vi "Picture Ring to Grid.vi"(11 "Selection Grid":T5) -> (1 "Valid":bool, 2 "Grid Summary":T4, 3 "Map":map{T1, T2}(c390))   [LabVIEW 2019, in "Grassfire Algorithm.lvclass"]
doc: "From the Start Grid of just the picture ring array, calculate where the start and end are."
uses:
  Grassfire Algorithm.lvclass
  Selection Grid Cell--array.ctl
  Selection--picture ring.ctl
  Grid Summary--cluster.ctl
  Index Column Row--cluster.ctl
  Solution Grid Cell Private--cluster.ctl
  Solution--picture ring.ctl
panel:
  out "1 End":bool
  out "1 Start":bool
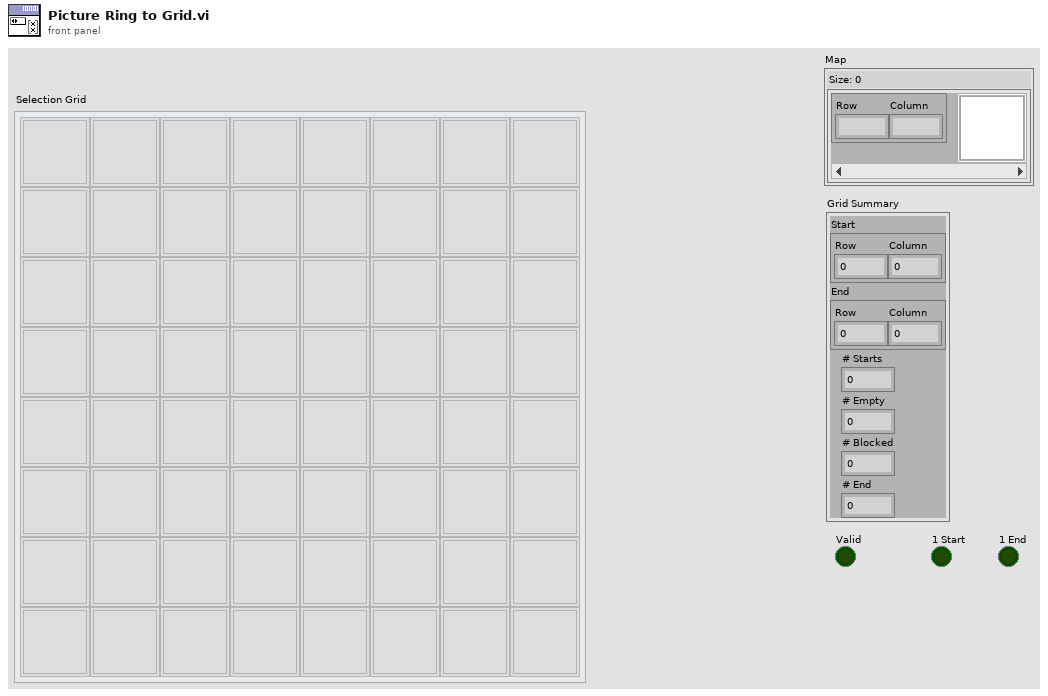
[diagram p1: front panel]
types:
  T1 = typedef "Grassfire Algorithm.lvclass/Index Column Row--cluster.ctl" = cluster{"Row":i32, "Column":i32}
  T2 = typedef "Grassfire Algorithm.lvclass/Solution Grid Cell Private--cluster.ctl" = cluster{"Picture":T3, "Value":dbl}
  T3 = typedef "Grassfire Algorithm.lvclass/Solution--picture ring.ctl" = i64
  T4 = typedef "Grassfire Algorithm.lvclass/Grid Summary--cluster.ctl" = cluster{"Start":T1, "End":T1, "# Starts":i32, "# Empty":i32, "# Blocked":i32, "# End":i32}
  T5 = typedef "Grassfire Algorithm.lvclass/Selection Grid Cell--array.ctl" = cluster{"Grid Value":T6}[][]
  T6 = typedef "Grassfire Algorithm.lvclass/Selection--picture ring.ctl" = i64
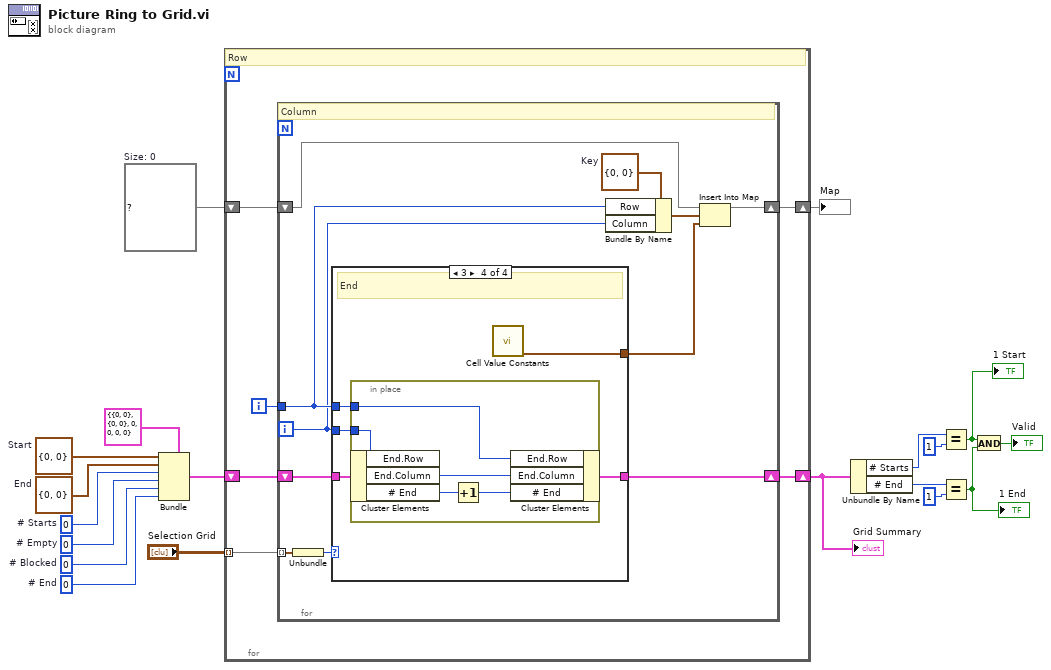
[diagram p0: block diagram]
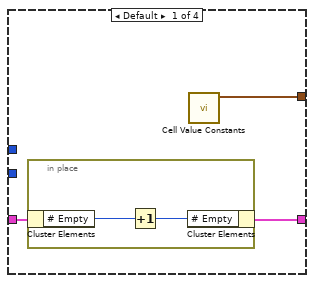
[diagram p2: hidden frame]
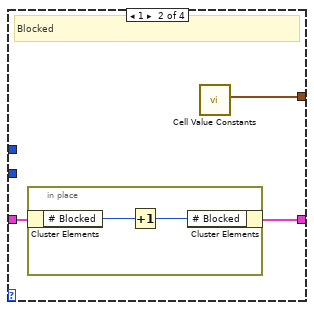
[diagram p3: hidden frame]
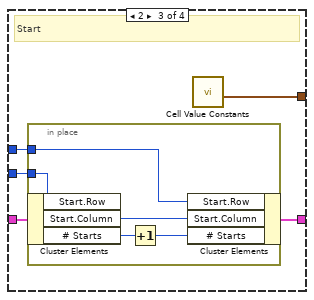
[diagram p4: hidden frame]
diagram:
  w2 = map{T1, T2} {}  # Size: 0
  w17 = T1 {"Row"=0, "Column"=0}  # End
  w13 = 0  # # End
  w14 = 0  # # Blocked
  w15 = 0  # # Empty
  w16 = 0  # # Starts
  w18 = T1 {"Row"=0, "Column"=0}  # Start
  n1 = Bundle(cluster=T4 {"Start"={"Row"=0, "Column"=0}, "End"={"Row"=0, "Column"=0}, "# Starts"=0, "# Empty"=0, "# Blocked"=0, "# End"=0} ("Grid Summary"), "Start"=w18, "End"=w17, "# Starts"=w16, "# Empty"=w15, "# Blocked"=w14, "# End"=w13) -> (w19:T4)
  n2 = for {
    tunnel: "Selection Grid" -> [w25] mode=indexing
    shift-right: [w23] -> w4
    shift-left: w19 -> [w24]
    shift-right: [w20] -> w1
    shift-left: w2 -> [w21]
    i -> [w22]
    # "Row"
    n3 = for {
      tunnel: w25 -> [w36] mode=indexing
      shift-right: [w34] -> w23
      shift-left: w24 -> [w35]
      tunnel: w22 -> [w29]
      shift-right: [w31] -> w20
      shift-left: w21 -> [w32]
      i -> [w28]
      w33 = T1 {"Row"=0, "Column"=0}  # Key
      # "Column"
      n4 = Unbundle(w36) -> ("Grid Value"=w26:T6)
      n5 = case shown="3" w26 {
        tunnel: w35 -> [w39 w44 w51 w60]
        tunnel: [w38 w43 w50 w59] -> w34
        tunnel: w29 -> [_ _ w49 w58]
        tunnel: w28 -> [_ _ w48 w57]
        tunnel: [w37 w42 w47 w56] -> w27
        frame Default {
          n6 = in-place {
            n7 = in-place-cluster #1(w39) -> ("# Empty"=w41:i32)
            n8 = Increment(x=w41) -> (x+1=w40:i32)
            n9 = in-place-cluster #1("# Empty"=w40) -> (w38:T4)
          }
          n10 = call "Cell Value Constants.vi"() -> ("Empty"=w37:T2)  [unwired: 8 in, 3 out]
        }
        frame 1 {
          # "Blocked"
          n11 = in-place {
            n12 = in-place-cluster #2(w44) -> ("# Blocked"=w46:i32)
            n13 = Increment(x=w46) -> (x+1=w45:i32)
            n14 = in-place-cluster #2("# Blocked"=w45) -> (w43:T4)
          }
          n15 = call "Cell Value Constants.vi"() -> ("Blocked"=w42:T2)  [unwired: 8 in, 3 out]
        }
        frame 2 {
          # "Start"
          n16 = in-place {
            in-place-border: w49 -> [w53]
            in-place-border: w48 -> [w52]
            n17 = in-place-cluster #3(w51) -> ("# Starts"=w55:i32)  [unwired: 2 out]
            n18 = Increment(x=w55) -> (x+1=w54:i32)
            n19 = in-place-cluster #3("Start.Row"=w53, "Start.Column"=w52, "# Starts"=w54) -> (w50:T4)
          }
          n20 = call "Cell Value Constants.vi"() -> ("Start"=w47:T2)  [unwired: 8 in, 3 out]
        }
        frame 3 {
          # "End"
          n21 = in-place {
            in-place-border: w58 -> [w62]
            in-place-border: w57 -> [w61]
            n22 = in-place-cluster #4(w60) -> ("# End"=w64:i32)  [unwired: 2 out]
            n23 = Increment(x=w64) -> (x+1=w63:i32)
            n24 = in-place-cluster #4("End.Row"=w62, "End.Column"=w61, "# End"=w63) -> (w59:T4)
          }
          n25 = call "Cell Value Constants.vi"() -> ("End"=w56:T2)  [unwired: 8 in, 3 out]
        }
      }
      n26 = Bundle By Name(cluster=w33, "Row"=w29, "Column"=w28) -> (w30:T1)
      n27 = Insert Into Map(map in=w32, key=w30, value=w27) -> (map out=w31:map{T1, T2})  [unwired: 2 out]
    }
  }
  "Grid Summary" <- w4
  "Map" <- w1
  n28 = Unbundle By Name(w4) -> ("# Starts"=w12:i32, "# End"=w9:i32)
  n29 = Equal?(x=w12, y=1) -> (x = y?=w8:bool)
  "1 Start" <- w8
  n30 = Equal?(x=w9, y=1) -> (x = y?=w6:bool)
  "1 End" <- w6
  n31 = And(x=w8, y=w6) -> (x .and. y?=→"Valid":bool)
